vi "GetEvtReports.vi"(8 "error in (no error)":errorcluster, 11 "UserEvtPlugins in":refnum<class "UserWfrmPlugins.lvclass">) -> (0 "error out":errorcluster, 3 "UserEvtPlugins out":refnum<class "UserWfrmPlugins.lvclass">)   [LabVIEW 2014, in "WfrmPlugins.lvlib" / "UserWfrmPlugins.lvclass"]
uses:
  UserWfrmPlugins.lvclass
  EventPluginBaseClass/TypeDefs/clEvtReport.ctl
  <vilib>/Utility/config.llb/Read Key (String).vi
  <vilib>/imath/engines/lvmath/Plug In/_Char/NIMS_CH_String to Character Array.vi
  C:/Labview Data/MathScriptVIs/MCStatic_33564263232_4d8935da10af67934e26c76271b4abc0.vi
  <instcachedir>/0/MCStatic_33564263232_4d8935da10af67934e26c76271b4abc0_C0A0904B4EAB49B78AB0B22F4FB46D70.lvgen/MCStatic_33564263232_4d8935da10af67934e26c76271b4abc0_C0A0904B4EAB49B78AB0B22F4FB46D70_000.vi
  <vilib>/imath/engines/lvmath2/RunTimeEngine/UserFunctionToken/NIMS_UserFunction_CondDefined.vi
  <instcachedir>/0/NIMS_UserFunction_CondDefined_359D6D699583402F98E5D4DB7FB40D41.lvgen/NIMS_UserFunction_CondDefined_359D6D699583402F98E5D4DB7FB40D41_000.vi
  <vilib>/imathl/engines/lvmath/Functions/Error Handling/Create Error.vi
  <instcachedir>/0/NIMS_UserFunction_CondDefined_359D6D699583402F98E5D4DB7FB40D41.lvgen/NIMS_UserFunction_CondDefined_359D6D699583402F98E5D4DB7FB40D41_003.vi
  <instcachedir>/0/NIMS_UserFunction_CondDefined_359D6D699583402F98E5D4DB7FB40D41.lvgen/NIMS_UserFunction_CondDefined_359D6D699583402F98E5D4DB7FB40D41_002.vi
  <instcachedir>/0/NIMS_UserFunction_CondDefined_359D6D699583402F98E5D4DB7FB40D41.lvgen/NIMS_UserFunction_CondDefined_359D6D699583402F98E5D4DB7FB40D41_001.vi
  <vilib>/imath/engines/lvmath2/RunTimeEngine/VariableToken/NIMS_VariableToken_CondDefined.vi
  <instcachedir>/0/NIMS_VariableToken_CondDefined_EE8DD211A89249938CE6537267F5C9B3.lvgen/NIMS_VariableToken_CondDefined_EE8DD211A89249938CE6537267F5C9B3_006.vi
  <instcachedir>/0/NIMS_VariableToken_CondDefined_EE8DD211A89249938CE6537267F5C9B3.lvgen/NIMS_VariableToken_CondDefined_EE8DD211A89249938CE6537267F5C9B3_001.vi
  <instcachedir>/0/NIMS_VariableToken_CondDefined_EE8DD211A89249938CE6537267F5C9B3.lvgen/NIMS_VariableToken_CondDefined_EE8DD211A89249938CE6537267F5C9B3_002.vi
  <instcachedir>/0/NIMS_VariableToken_CondDefined_EE8DD211A89249938CE6537267F5C9B3.lvgen/NIMS_VariableToken_CondDefined_EE8DD211A89249938CE6537267F5C9B3_004.vi
  <vilib>/imath/engines/lvmath2/RunTimeEngine/NodeEndStatement/NIMS_NodeEndStatement_Get Vector.vi
  <instcachedir>/0/NIMS_NodeEndStatement_Get Vector_00D1625602D843AD9D7EC134A9EC13A2.lvgen/NIMS_NodeEndStatement_Get Vector_00D1625602D843AD9D7EC134A9EC13A2_002.vi
  <instcachedir>/0/NIMS_NodeEndStatement_Get Vector_00D1625602D843AD9D7EC134A9EC13A2.lvgen/NIMS_NodeEndStatement_Get Vector_00D1625602D843AD9D7EC134A9EC13A2_001.vi
  <vilib>/imath/engines/lvmath/Functions/Error Handling/MergeErrorsWrapper.vi
  <vilib>/imath/engines/lvmath2/RunTimeEngine/NodeEndStatement/NIMS_NodeEndStatement_Output.vi
  <instcachedir>/0/NIMS_NodeEndStatement_Output_53EC0D466D134D7ABD903AC30B43404B.lvgen/NIMS_NodeEndStatement_Output_53EC0D466D134D7ABD903AC30B43404B_005.vi
  <instcachedir>/0/NIMS_NodeEndStatement_Output_53EC0D466D134D7ABD903AC30B43404B.lvgen/NIMS_NodeEndStatement_Output_53EC0D466D134D7ABD903AC30B43404B_003.vi
  <vilib>/imath/engines/lvmath2/RunTimeEngine/ErrorHandling/NIMS_Finalize Error.vi
  Matlab/User/UserEvtRptWrapper.m
  Matlab/User/Harm60255Rpt.m
  Matlab/User/userfunc1.m
  Matlab/User/userfunc2.m
  <vilib>/Utility/config.llb/NI_LVConfig.lvlib
  EventPluginBaseClass/BaseWfrmPlugin.lvclass
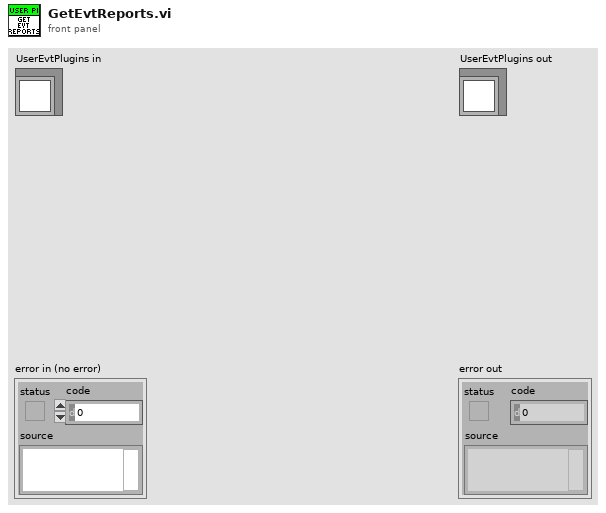
[diagram p1: front panel]
types:
  T1 = typedef "WfrmPlugins.lvlib/BaseWfrmPlugin.lvclass/clEvtReport.ctl" = cluster{"Timestamp":dbl, "Synx":cdb[], "Freq":dbl, "ROCOF":dbl}
  T2 = typedef "WfrmPlugins.lvlib/BaseWfrmPlugin.lvclass/WfrmConfig.ctl" = cluster{"T0(UTC)":dbl, "F0":dbl, "Fs":i32, "FSamp":u32}
  T3 = typedef "NI_LVConfig.lvlib/Config Data RefNum.ctl" = refnum<k1>
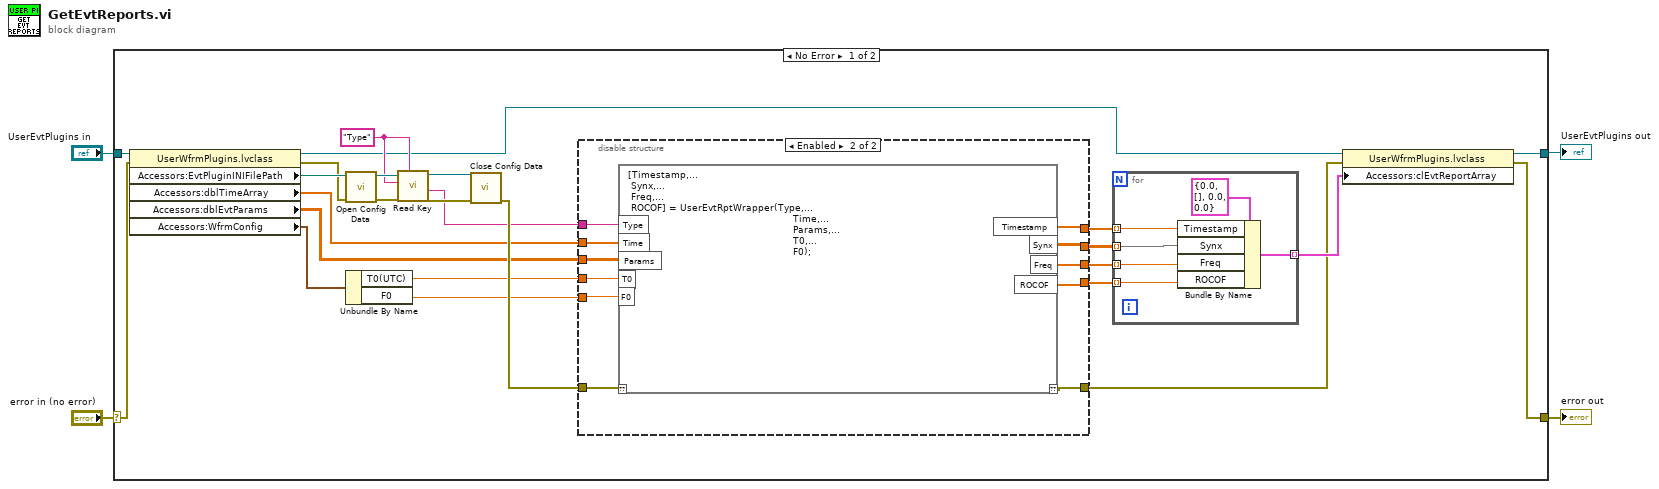
[diagram p0: block diagram]
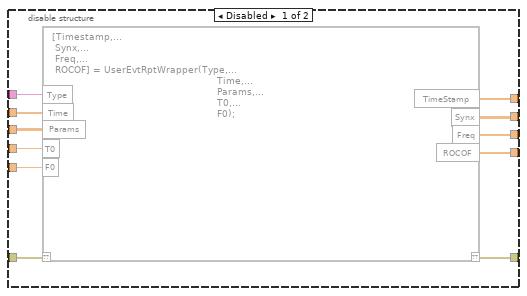
[diagram p2: hidden frame]
diagram:
  n1 = case shown="No Error" "error in (no error)" {
    selector: "error in (no error)" -> [w28 w198]
    tunnel: [w12 w198] -> w1
    tunnel: [w13 w197] -> w2
    tunnel: "UserEvtPlugins in" -> [w29 w197]
    frame No Error {
      w23 = "Type" ("section")
      n2 = property class="UserWfrmPlugins.lvclass"(reference=w29, error in=w28) -> (reference out=w5:refnum<class "UserWfrmPlugins.lvclass">, error out=w26:errorcluster, "Accessors:EvtPluginINIFilePath"=w27:path, "Accessors:dblTimeArray"=w18:dbl[], "Accessors:dblEvtParams"=w17:dbl[][], "Accessors:WfrmConfig"=w16:T2)
      n3 = call <vilib>:"Open Config Data.vi"("error in (no error)"=w26, "configuration file path"=w27) -> ("error out"=w25:errorcluster, "refnum"=w24:T3)  [unwired: 7 in, 1 out]
      n4 = Unbundle By Name(w16) -> ("T0(UTC)"=w15:dbl, "F0"=w14:dbl)
      n5 = call-poly <vilib>:"Read Key.vi"("section"=w23, "error in (no error)"=w25, "key"=w23, "refnum"=w24) -> ("error out"=w21:errorcluster, "value"=w19:string, "refnum out"=w22:T3)  [unwired: 4 in, 1 out]
      n6 = call <vilib>:"Close Config Data.vi"("error in (no error)"=w21, "refnum"=w22) -> ("error out"=w20:errorcluster)  [unwired: 8 in, 1 out]
      n7 = disable-structure shown="Enabled" {
        disable-tunnel: w20 -> [w40 w51]
        disable-tunnel: w19 -> [w39 w49]
        disable-tunnel: w18 -> [w38 w48]
        disable-tunnel: w17 -> [w37 w47]
        disable-tunnel: w15 -> [w36 w46]
        disable-tunnel: w14 -> [w35 w45]
        disable-tunnel: [w34 w44] -> w11
        disable-tunnel: [w33 w43] -> w10
        disable-tunnel: [w30 w42] -> w9
        disable-tunnel: [w32 w41] -> w8
        disable-tunnel: [w31 w50] -> w6
        frame Disabled {
          n8 = script code="[Timestamp,...\n Synx,...\n Freq,...\n ROCOF] = UserEvtRptWrapper(Type,...\n                                                       Time,...\n                                                       Params,...\n                                                       T0,...\n                                                       F0);"("??"=w40, "Type"=w39, "Time"=w38, "Params"=w37, "T0"=w36, "F0"=w35) -> ("??"=w31:errorcluster, "TimeStamp"=w34:dbl[], "Synx"=w33:cdb[][], "Freq"=w30:dbl[], "ROCOF"=w32:dbl[])
        }
        frame Enabled {
          n9 = mathscript code="[Timestamp,...\n Synx,...\n Freq,...\n ROCOF] = UserEvtRptWrapper(Type,...\n                                                       Time,...\n                                                       Params,...\n                                                       T0,...\n                                                       F0);"("??"=w51, "Type"=w49, "Time"=w48, "Params"=w47, "T0"=w46, "F0"=w45) -> ("??"=w50:errorcluster, "Timestamp"=w44:dbl[], "Synx"=w43:cdb[][], "Freq"=w42:dbl[], "ROCOF"=w41:dbl[])
        }
      }
      n10 = for {
        tunnel: w11 -> [w195] mode=indexing
        tunnel: w10 -> [w194] mode=indexing
        tunnel: w9 -> [w193] mode=indexing
        tunnel: w8 -> [w192] mode=indexing
        tunnel: [w191] -> w7 mode=indexing
        n11 = Bundle By Name(cluster=T1 {"Timestamp"=0.0, "Synx"=[], "Freq"=0.0, "ROCOF"=0.0} ("clEvtReport"), "Timestamp"=w195, "Synx"=w194, "Freq"=w193, "ROCOF"=w192) -> (w191:T1)
      }
      n12 = property class="UserWfrmPlugins.lvclass"(reference=w5, error in=w6, "Accessors:clEvtReportArray"=w7) -> (reference out=w13:refnum<class "UserWfrmPlugins.lvclass">, error out=w12:errorcluster)
    }
    frame Error {
    }
  }
  "error out" <- w1
  "UserEvtPlugins out" <- w2
